vi "5492_AutonomousStraightVision.vi"(7 "Length":dbl=3000.0, 8 "Margin of Error (Pixels)":i32=20, 9 "Pixel Height Goal":dbl=2400.0 format="%#_13g", 10 "RobotDriveDevRef":T1={"DevStatus"={"status"=FALSE, "code"=0, "source"=""}, "Motors[]"=[], "Square Inputs"=FALSE, "Max Output"=1.0}) -> (3 "RobotDriveDevRef":T1={"DevStatus"={"status"=FALSE, "code"=0, "source"=""}, "Motors[]"=[], "Square Inputs"=FALSE, "Max Output"=1.0})   [LabVIEW 2016]
uses:
  <vilib>/Rock Robotics/WPI/RobotDrive/WPI_RobotDriveDevRef.ctl
  <vilib>/Rock Robotics/WPI/MotorControl/WPI_MotorControlDeviceRef.ctl
  <vilib>/Rock Robotics/WPI/MotorControl/WPI_MotorControlType.ctl
  <vilib>/Rock Robotics/SystemInterfaces/DIO/FPGA_DIOPWMChannel.ctl
  <vilib>/Rock Robotics/WPI/PWM/WPI_PWMDeadband.ctl
  5492_WPI_RobotDriveMotorSelectorEnum.ctl
  <vilib>/Rock Robotics/WPI/RobotDrive/WPI_RobotDriveSafetyCheck.vi
panel:
  out "Numeric":i32
  out "Motor Output 2":dbl
  out "Motor Output":dbl
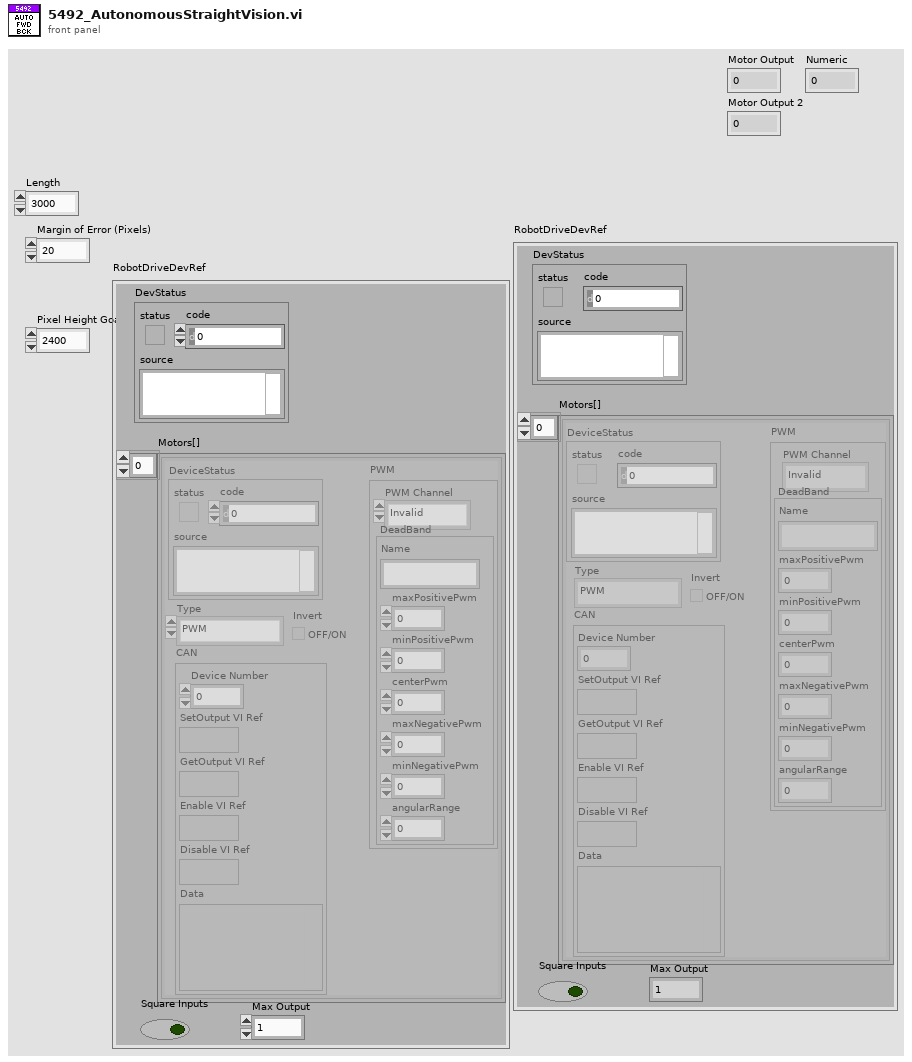
[diagram p1: front panel]
types:
  T1 = typedef "WPI_RobotDriveDevRef.ctl" = cluster{"DevStatus":errorcluster, "Motors[]":T2[], "Square Inputs":bool, "Max Output":dbl}
  T2 = typedef "WPI_MotorControlDeviceRef.ctl" = cluster{"DeviceStatus":errorcluster, "Type":T3, "PWM":cluster{"PWM Channel":T4, "DeadBand":T5}, "CAN":cluster{"Device Number":u8, "SetOutput VI Ref":variant, "GetOutput VI Ref":variant, "Enable VI Ref":variant, "Disable VI Ref":variant, "Data":variant}, "Invert":bool}
  T3 = typedef "WPI_MotorControlType.ctl" = enum16{"PWM", "CAN"}
  T4 = typedef "FPGA_DIOPWMChannel.ctl" = enum8{"PWM 0", "PWM 1", "PWM 2", "PWM 3", "PWM 4", "PWM 5", "PWM 6", "PWM 7", "PWM 8", "PWM 9", "PWM MXP 0", "PWM MXP 1", "PWM MXP 2", "PWM MXP 3", "PWM MXP 4", "PWM MXP 5", "PWM MXP 6", "PWM MXP 7", "PWM MXP 8", "PWM MXP 9", "Invalid"}
  T5 = typedef "WPI_PWMDeadband.ctl" = cluster{"Name":string, "maxPositivePwm":i32, "minPositivePwm":i32, "centerPwm":i32, "maxNegativePwm":i32, "minNegativePwm":i32, "angularRange":u16}
  T6 = typedef "5492_WPI_RobotDriveMotorSelectorEnum.ctl" = enum16{"Front left motor", "Front right motor", "Back left motor", "Back right motor"}
  T7 = typedef "WPI_CANTalonSRX_GlobalStatus.ctl" = cluster{"Applied Throttle":dbl, "Module Enabled":bool, "CAN Error":errorcluster, "Closed Loop Error":dbl, "Forward Limit Switch Closed":bool, "Reverse Limit Switch Closed":bool, "Sensor Position":dbl, "Sensor Velocity":dbl, "Current":dbl, "Sticky Fault - Over Temp":bool, "Sticky Fault - Under Voltage":bool, "Sticky Fault - Forward Limit":bool, "Sticky Fault - Reverse Limit":bool, "Sticky Fault - Forward Soft Limit":bool, "Sticky Fault - Reverse Soft Limit":bool, "Brake is Enabled":bool, "Encoder Position":dbl, "Encoder Velocity":dbl, "Encoder Index Count":dbl, "Encoder A Pin State":bool, "Encoder B Pin State":bool, "Encoder Index Pin State":bool, "Analog In":dbl, "Analog In Velocity":dbl, "Temperature (C)":dbl, "Battery Voltage":dbl, "Control 5 Is Supported":bool, "Current Profile Slot Select":dbl, "Pos Div 8":bool, "Vel Div 4":bool, "Pulse Width Position":i32, "Pulse Width Velocity":i32, "Pulse Width Rise To Rise (us)":i32, "Pulse Width Rise To Fall (us)":i32, "Mot Prof Active Is Under Run":bool, "Mot Prof Active Has Under Run":bool, "Mot Prof Active Is Last":bool, "Mot Prof Active Velocity Only":bool, "Mot Prof Active Is Valid":bool, "Mot Prof Buffer Is Full":bool, "Mot Prof Active Profile Slot Select":i32, "Mot Prof NextID":i32, "Mot Prof Count":i32, "Mot Prof Active Velocity":dbl, "Mot Prof Active Position":dbl, "Mot Prof Output Enable":i32}
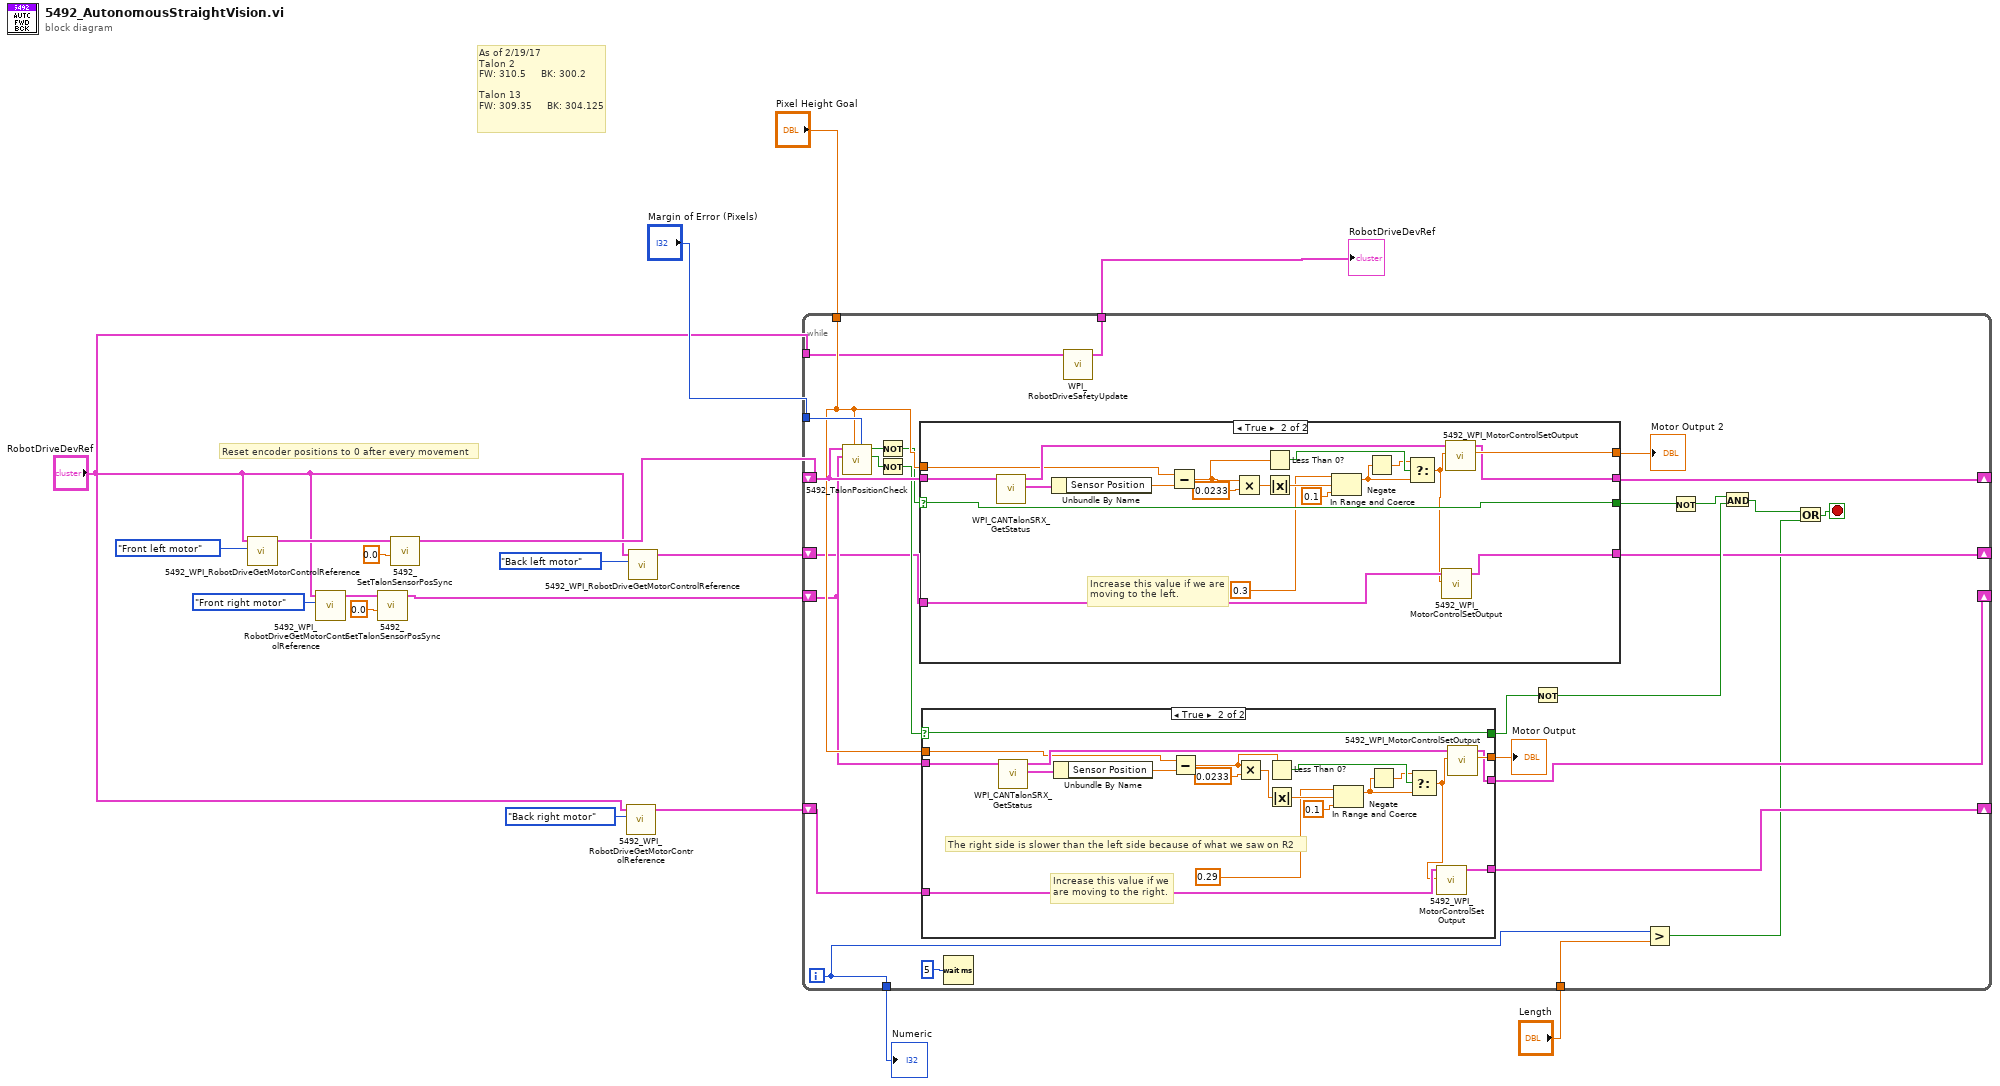
[diagram p0: block diagram]
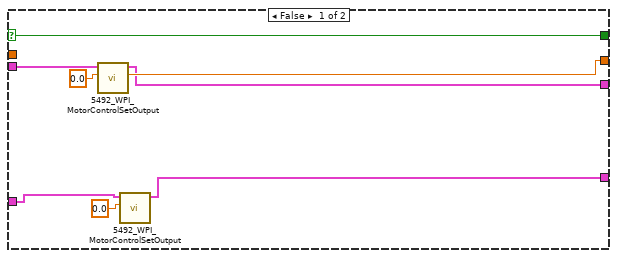
[diagram p2: hidden frame]
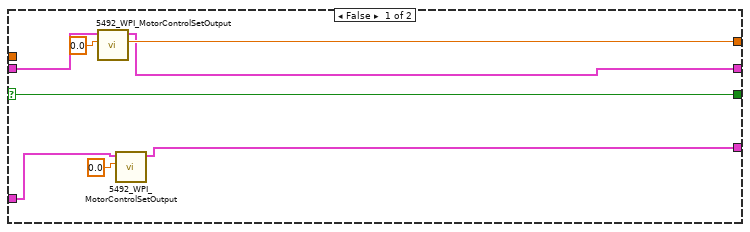
[diagram p3: hidden frame]
diagram:
  # "As of 2/19/17\nTalon 2 \nFW: 310.5     BK: 300.2\n\nTalon 13\nFW: 309.35     BK: 304.125"
  # "Reset encoder positions to 0 after every movement"
  n1 = call "5492_WPI_RobotDriveGetMotorControlReference.vi"("MotorIndex"=5492_WPI_RobotDriveMotorSelectorEnum."Front left motor", "RobotDriveDevRef"="RobotDriveDevRef") -> ("MotorControlDeviceRef"=w13:T2)  [unwired: 9 out]
  n2 = call "5492_WPI_RobotDriveGetMotorControlReference.vi"("MotorIndex"=5492_WPI_RobotDriveMotorSelectorEnum."Front right motor", "RobotDriveDevRef"="RobotDriveDevRef") -> ("MotorControlDeviceRef"=w10:T2)  [unwired: 9 out]
  n3 = call "5492_SetTalonSensorPosSync.vi"("Pos"=0.0 ("New Sensor Position"), "CAN Talon SRX Ref In"=w10) -> ("CAN Talon SRX Ref Out"=w9:T2)  [unwired: 8 in, 1 out]
  n4 = call "5492_SetTalonSensorPosSync.vi"("Pos"=0.0 ("New Sensor Position"), "CAN Talon SRX Ref In"=w13) -> ("CAN Talon SRX Ref Out"=w12:T2)  [unwired: 8 in, 1 out]
  n5 = call "5492_WPI_RobotDriveGetMotorControlReference.vi"("MotorIndex"=5492_WPI_RobotDriveMotorSelectorEnum."Back right motor", "RobotDriveDevRef"="RobotDriveDevRef") -> ("MotorControlDeviceRef"=w5:T2)  [unwired: 9 out]
  n6 = call "5492_WPI_RobotDriveGetMotorControlReference.vi"("MotorIndex"=5492_WPI_RobotDriveMotorSelectorEnum."Back left motor", "RobotDriveDevRef"="RobotDriveDevRef") -> ("MotorControlDeviceRef"=w6:T2)  [unwired: 9 out]
  n7 = while {
    tunnel: "Pixel Height Goal" -> [w43]
    tunnel: "Margin of Error (Pixels)" -> [w44]
    shift-right: [w31] -> _
    shift-left: w12 -> [w45]
    shift-right: [w30] -> _
    shift-left: w9 -> [w42]
    tunnel: [w23] -> w15
    shift-right: [w28] -> _
    shift-left: w6 -> [w29]
    shift-right: [w26] -> _
    shift-left: w5 -> [w27]
    tunnel: [w25] -> w4
    tunnel: "RobotDriveDevRef" -> [w24]
    tunnel: "Length" -> [w22]
    i -> [w23]
    stop <- w21 stop-if-true
    n8 = call "5492_TalonPositionCheck.vi"("Margin of Error"=w44, "Position Goal"=w43, "CAN Talon SRX Ref Right"=w42, "CAN Talon SRX Ref Left"=w45) -> ("RIght Achieved"=w41:bool, "Left Achieved"=w39:bool)  [unwired: 6 in]
    n9 = Not(x=w39) -> (.not. x?=w38:bool)
    n10 = Not(x=w41) -> (.not. x?=w40:bool)
    n11 = case shown="True" w38 {
      selector: w38 -> [w80 w92]
      tunnel: w45 -> [w82 w102]
      tunnel: w43 -> [_ w93]
      tunnel: [w80 w92] -> w34
      tunnel: [w79 w91] -> w36
      tunnel: [w78 w90] -> w31
      tunnel: w29 -> [w76 w88]
      tunnel: [w75 w87] -> w28
      frame False {
        n12 = call "5492_WPI_MotorControlSetOutput.vi"("Output"=0.0 ("P"), "MotorControlDevRef"=w82) -> ("Motor Output"=w79:dbl, "MotorControlDevRef"=w78:T2)  [unwired: 7 in, 1 out]
        n13 = call "5492_WPI_MotorControlSetOutput.vi"("Output"=0.0 ("P"), "MotorControlDevRef"=w76) -> ("MotorControlDevRef"=w75:T2)  [unwired: 7 in, 2 out]
      }
      frame True {
        # "Increase this value if we are\nmoving to the left."
        n14 = call <vilib>:"WPI_CANTalonSRX_GetStatus.vi"("CAN Talon SRX Ref"=w102) -> ("Talon SRX Status"=w89:T7, "CAN Talon SRX Ref"=w94:T2)  [unwired: 8 in, 1 out]
        n15 = Unbundle By Name(w89) -> ("Sensor Position"=w85:dbl)
        n16 = Subtract(x=w93, y=w85) -> (x-y=w84:dbl)
        n17 = Multiply(x=w84, y=0.0233) -> (x*y=w95:dbl)
        n18 = Less Than 0?(x=w84) -> (x < 0?=w99:bool)
        n19 = Absolute Value(x=w95) -> (abs(x)=w96:dbl)
        n20 = In Range and Coerce(upper limit=0.3 ("f"), x=w96, lower limit=0.1) -> (coerced(x)=w97:dbl)  [unwired: 1 out]
        n21 = Negate(x=w97) -> (-x=w98:dbl)
        n22 = Select(t=w98, s=w99, f=w97) -> (s? t:f=w86:dbl)
        n23 = call "5492_WPI_MotorControlSetOutput.vi"("Output"=w86, "MotorControlDevRef"=w88) -> ("MotorControlDevRef"=w87:T2)  [unwired: 7 in, 2 out]
        n24 = call "5492_WPI_MotorControlSetOutput.vi"("Output"=w86, "MotorControlDevRef"=w94) -> ("Motor Output"=w91:dbl, "MotorControlDevRef"=w90:T2)  [unwired: 7 in, 1 out]
      }
    }
    "Motor Output 2" <- w36
    n25 = case shown="True" w40 {
      selector: w40 -> [w52 w64]
      tunnel: w42 -> [w53 w74]
      tunnel: w43 -> [_ w65]
      tunnel: [w52 w64] -> w35
      tunnel: [w51 w63] -> w37
      tunnel: [w50 w62] -> w30
      tunnel: w27 -> [w49 w60]
      tunnel: [w48 w59] -> w26
      frame False {
        n26 = call "5492_WPI_MotorControlSetOutput.vi"("Output"=0.0 ("P"), "MotorControlDevRef"=w53) -> ("Motor Output"=w51:dbl, "MotorControlDevRef"=w50:T2)  [unwired: 7 in, 1 out]
        n27 = call "5492_WPI_MotorControlSetOutput.vi"("Output"=0.0 ("P"), "MotorControlDevRef"=w49) -> ("MotorControlDevRef"=w48:T2)  [unwired: 7 in, 2 out]
      }
      frame True {
        # "Increase this value if we\nare moving to the right."
        # "The right side is slower than the left side because of what we saw on R2"
        n28 = call <vilib>:"WPI_CANTalonSRX_GetStatus.vi"("CAN Talon SRX Ref"=w74) -> ("Talon SRX Status"=w61:T7, "CAN Talon SRX Ref"=w66:T2)  [unwired: 8 in, 1 out]
        n29 = Unbundle By Name(w61) -> ("Sensor Position"=w57:dbl)
        n30 = Subtract(x=w65, y=w57) -> (x-y=w56:dbl)
        n31 = Multiply(x=w56, y=0.0233) -> (x*y=w67:dbl)
        n32 = Less Than 0?(x=w56) -> (x < 0?=w71:bool)
        n33 = Absolute Value(x=w67) -> (abs(x)=w68:dbl)
        n34 = In Range and Coerce(upper limit=0.29 ("f"), x=w68, lower limit=0.1) -> (coerced(x)=w69:dbl)  [unwired: 1 out]
        n35 = Negate(x=w69) -> (-x=w70:dbl)
        n36 = Select(t=w70, s=w71, f=w69) -> (s? t:f=w58:dbl)
        n37 = call "5492_WPI_MotorControlSetOutput.vi"("Output"=w58, "MotorControlDevRef"=w60) -> ("MotorControlDevRef"=w59:T2)  [unwired: 7 in, 2 out]
        n38 = call "5492_WPI_MotorControlSetOutput.vi"("Output"=w58, "MotorControlDevRef"=w66) -> ("Motor Output"=w63:dbl, "MotorControlDevRef"=w62:T2)  [unwired: 7 in, 1 out]
      }
    }
    "Motor Output" <- w37
    n39 = Wait (ms)(milliseconds to wait=u32 5) -> ()  [unwired: 1 out]
    n40 = call <vilib>:"WPI_RobotDriveSafetyUpdate.vi"("RobotDriveDevRef"=w24) -> ("RobotDriveDevRef"=w25:T1)  [unwired: 1 in, 9 out]
    n41 = Not(x=w35) -> (.not. x?=w33:bool)
    n42 = Greater?(x=w23, y=w22) -> (0:w19:bool)
    n43 = Not(x=w34) -> (.not. x?=w32:bool)
    n44 = And(x=w32, y=w33) -> (x .and. y?=w20:bool)
    n45 = Or(x=w20, y=w19) -> (x .or. y?=w21:bool)
  }
  "RobotDriveDevRef" <- w4
  "Numeric" <- w15
